vi "file add 1D data.vi"(10 "element":dbl[](array[numeric]), 11 "file path (dialog if empty)":path) -> ()   [LabVIEW 2016]
uses:
  <vilib>/Utility/file.llb/Read Delimited Spreadsheet (DBL).vi
  <vilib>/Utility/file.llb/Write Delimited Spreadsheet (DBL).vi
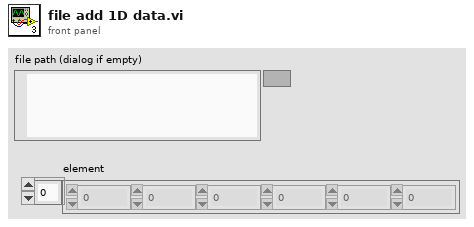
[diagram p1: front panel]
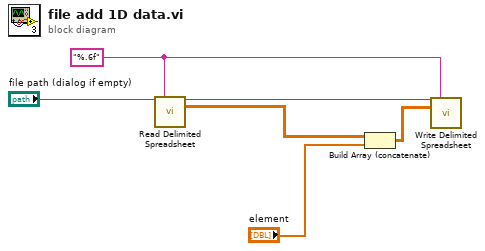
[diagram p0: block diagram]
diagram:
  w1 = "%.6f" ("format (%.3f)")
  n1 = call-poly <vilib>:"Read Delimited Spreadsheet.vi"("file path (dialog if empty)"="file path (dialog if empty)", "format (%.3f)"=w1) -> ("new file path (Not A Path if cancelled)"=w4:path, "all rows"=w6:dbl[][])  [unwired: 8 in, 4 out]
  n2 = Build Array (concatenate)(w6, "element") -> (w5:dbl[][])
  n3 = call-poly <vilib>:"Write Delimited Spreadsheet.vi"("file path (dialog if empty)"=w4, "format (%.3f)"=w1, "2D data"=w5) -> ()  [unwired: 11 in, 2 out]
